vi "2_1_LV23.vi"() -> ()   [LabVIEW 2023, in "2025.lvlib"]
uses:
  2025.lvlib
  <vilib>/Analysis/NI_AALBase.lvlib
  <vilib>/Analysis/1siggen.llb/Ramp Pattern by Delta.vi
  Program Files/National Instruments/LabVIEW 2025/user.lib/_OpenG.lib/string/string.llb/openg_string.lvlib
  Program Files/National Instruments/LabVIEW 2025/user.lib/_OpenG.lib/string/string.llb/Trim Whitespace (String Array)__ogtk.vi
panel:
  out "size(s)":i32
  out "Numeric":i32
  out "sum 2":u64
  out "number 2":u64[](array[numeric])
  out "Array 2":string[](array[string])
  out "output 7":string
  out "String out":string[](array[string])
  out "output 4":string
  out "output 3":string
  in  "Boolean":bool
  out "sum":u64
  out "number":u64[](array[numeric])
  out "Array":string[](array[string])
  out "substring 2":string
  out "substring":string
  out "length":i32
  out "decimal integer string":string[](array[string])
  out "Ramp Pattern":u64[](array[numeric])
  out "output 2":i32
  out "output 1":i32
  out "array":string[](array[string])
  # "1736195310 too LOW"
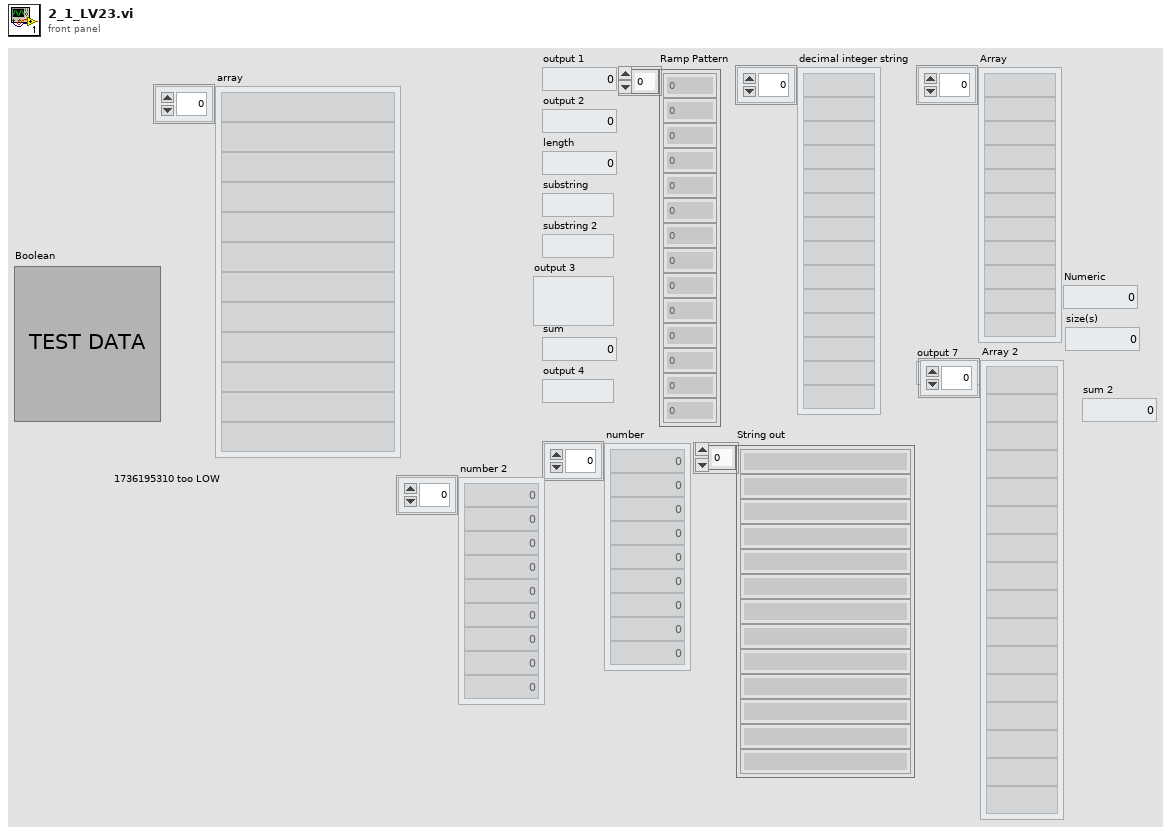
[diagram p1: front panel]
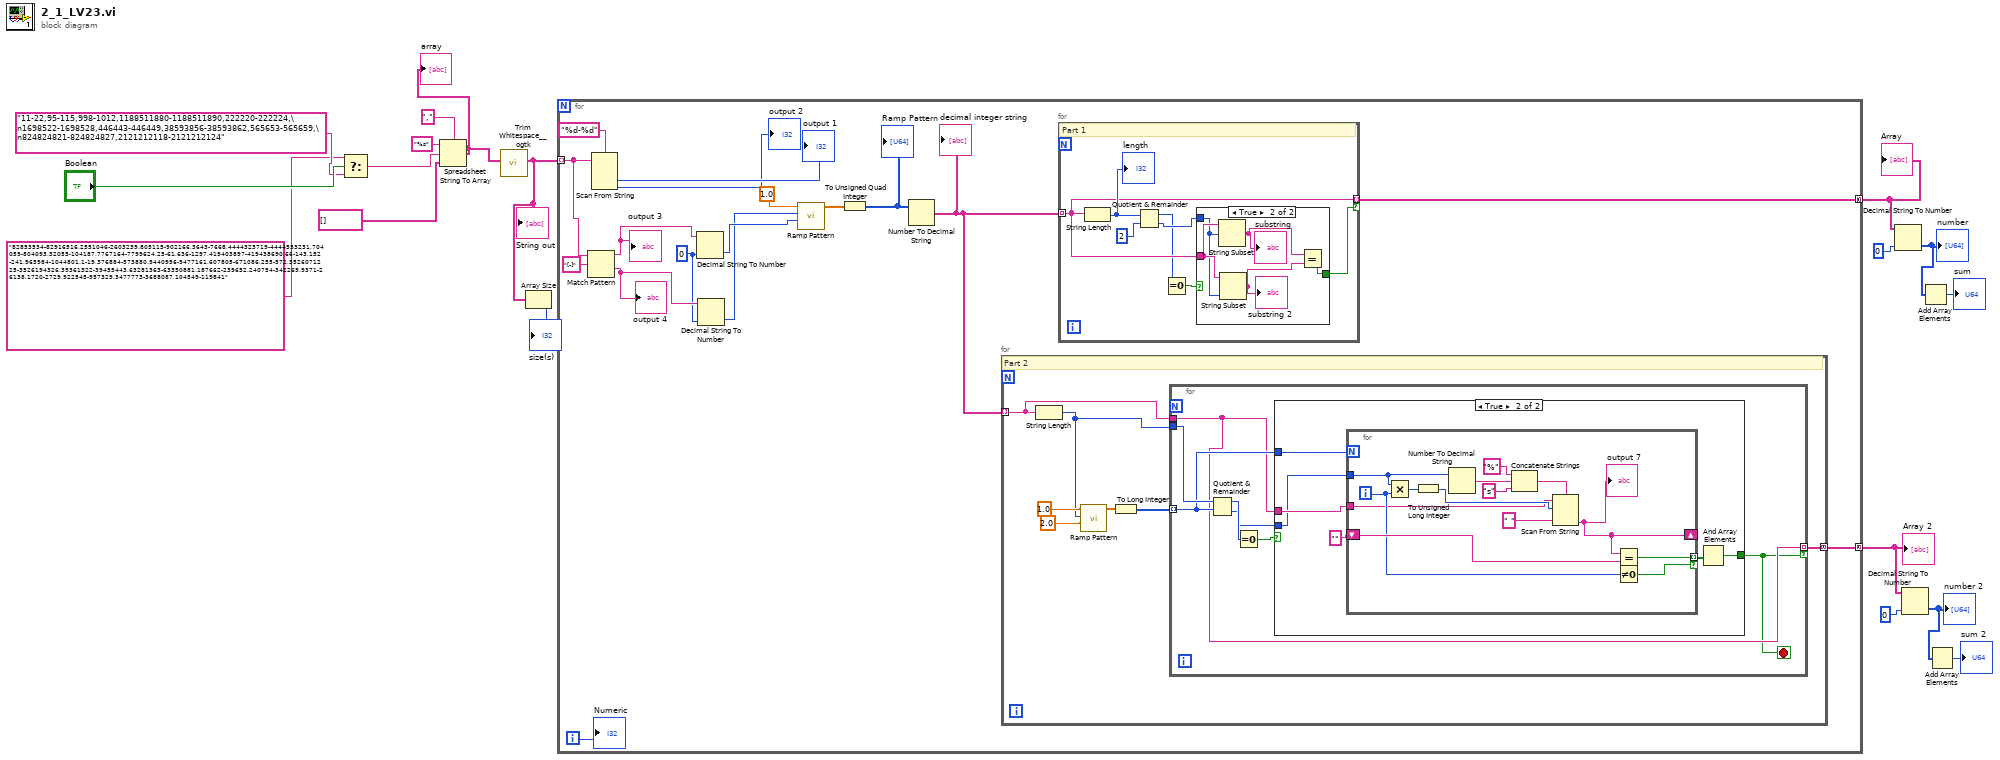
[diagram p0: block diagram]
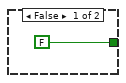
[diagram p3: hidden frame]
diagram:
  n1 = Select(t="82853534-82916516,2551046-2603239,805115-902166,3643-7668,4444323719-4444553231,704059-804093,32055-104187,7767164-7799624,25-61,636-1297,419403897-419438690,66-143,152-241,965984-1044801,1-19,376884-573880,9440956-9477161,607805-671086,255-572,3526071225-3526194326,39361322-39455443,63281363-63350881,187662-239652,240754-342269,9371-26138,1720-2729,922545-957329,3477773-3688087,104549-119841", s="Boolean", f="11-22,95-115,998-1012,1188511880-1188511890,222220-222224,\n1698522-1698528,446443-446449,38593856-38593862,565653-565659,\n824824821-824824827,2121212118-2121212124") -> (s? t:f=w8:string)
  n2 = Spreadsheet String To Array(delimiter (Tab)=",", format string="%s", spreadsheet string=w8, array type (2D Dbl)=string[] []) -> (array=w7:string[])
  "array" <- w7
  n3 = call-poly "Trim Whitespace__ogtk.vi"("String in"=w7) -> ("String out"=w2:string[])  [unwired: 6 in]
  "String out" <- w2
  n4 = Array Size(array=w2) -> (size(s)=→"size(s)":i32)
  n5 = for {
    tunnel: w2 -> [w28] mode=indexing
    tunnel: [w31] -> w15 mode=concatenating
    tunnel: [w20] -> w3 mode=concatenating
    i -> [w19]
    w24 = u64 0 ("default (0 I32)")
    n6 = Match Pattern(string=w28, regular expression="[-]") -> (before substring=w26:string, after substring=w25:string)  [unwired: 1 in, 2 out]
    "output 3" <- w26
    "output 4" <- w25
    n7 = Scan From String(format string="%d-%d", input string=w28) -> (output 1=→"output 1":i32, output 2=→"output 2":i32)  [unwired: 4 in, 3 out]
    n8 = Decimal String To Number(string=w26, default (0L)=w24) -> (number=w23:u64)  [unwired: 1 in, 1 out]
    n9 = Decimal String To Number(string=w25, default (0L)=w24) -> (number=w22:u64)  [unwired: 1 in, 1 out]
    n10 = call-poly <vilib>:"Ramp Pattern.vi"("start"=w23, "end"=w22, "delta"=1.0) -> ("Ramp Pattern"=w33:dbl[])  [unwired: 6 in, 2 out]
    n11 = To Unsigned Quad Integer(1:w33) -> (0:w32:u64[])
    "Ramp Pattern" <- w32
    n12 = Number To Decimal String(number=w32) -> (decimal integer string=w21:string[])  [unwired: 1 in]
    "decimal integer string" <- w21
    n13 = for {
      tunnel: w21 -> [w38] mode=indexing
      tunnel: [w36] -> w20 mode=concatenating
      # "Part 2"
      n14 = String Length(string=w38) -> (length=w37:i32)
      n15 = call-poly <vilib>:"Ramp Pattern.vi"("start"=2.0, "end"=w37, "delta"=1.0) -> ("Ramp Pattern"=w40:dbl[])  [unwired: 6 in, 2 out]
      n16 = To Long Integer(number=w40) -> (32bit integer=w39:i32[])
      n17 = for {
        tunnel: w39 -> [w45] mode=indexing
        tunnel: w38 -> [w44]
        tunnel: w37 -> [w49]
        tunnel: [w44] -> w36 mode=indexing if=w43
        stop <- w43 stop-if-true
        n18 = Quotient & Remainder(x=w49, y=w45) -> (x-y*floor(x/y)=w47:i32, floor(x/y)=w46:i32)
        n19 = Equal To 0?(x=w47) -> (x = 0?=w48:bool)
        n20 = case shown="True" w48 {
          tunnel: w46 -> [_ w54]
          tunnel: w44 -> [_ w55]
          tunnel: w45 -> [_ w53]
          tunnel: [_ w50] -> w43
          frame False {
          }
          frame True {
            n21 = for {
              N: w53 -> [_]
              tunnel: w54 -> [w62]
              tunnel: w55 -> [w56]
              shift-right: [w61] -> _
              shift-left: "" ("format string") -> [w60]
              tunnel: [w58] -> w51 mode=indexing if=w57
              i -> [w59]
              n22 = Multiply(x=w62, y=w59) -> (x*y=w69:i32)
              n23 = To Unsigned Long Integer(number=w69) -> (unsigned 32bit integer=w64:u32)
              n24 = Number To Decimal String(number=w62) -> (decimal integer string=w65:string)  [unwired: 1 in]
              n25 = Concatenate Strings("%" ("format string"), w65, "s" ("format string")) -> (w68:string)
              n26 = Scan From String(format string=w68, input string=w56, initial scan location=w64, default 1=" " ("format string")) -> (output 1=w61:string)  [unwired: 1 in, 3 out]
              "output 7" <- w61
              n27 = Equal?(x=w61, y=w60) -> (x = y?=w58:bool)
              n28 = Not Equal To 0?(x=w59) -> (x != 0?=w57:bool)
            }
            n29 = And Array Elements(Boolean array=w51) -> (logical AND=w50:bool)
          }
        }
      }
    }
    n30 = for {
      tunnel: w21 -> [w74] mode=indexing
      tunnel: [w74] -> w31 mode=indexing if=w72
      # "Part 1"
      n31 = String Length(string=w74) -> (length=w75:i32)
      "length" <- w75
      n32 = Quotient & Remainder(x=w75, y=2) -> (x-y*floor(x/y)=w70:i32, floor(x/y)=w71:i32)
      n33 = Equal To 0?(x=w70) -> (x = 0?=w73:bool)
      n34 = case shown="True" w73 {
        tunnel: w74 -> [_ w82]
        tunnel: w71 -> [_ w81]
        tunnel: [FALSE w78] -> w72
        frame False {
        }
        frame True {
          n35 = String Subset(string=w82, offset (0)=w81) -> (substring=w80:string)  [unwired: 1 in]
          "substring" <- w80
          n36 = String Subset(string=w82, length (rest)=w81) -> (substring=w79:string)  [unwired: 1 in]
          "substring 2" <- w79
          n37 = Equal?(x=w80, y=w79) -> (x = y?=w78:bool)
        }
      }
    }
    "Numeric" <- w19
  }
  "Array" <- w15
  "Array 2" <- w3
  n38 = Decimal String To Number(string=w15, default (0L)=u64 0 ("default (0 I32)")) -> (number=w14:u64[])  [unwired: 1 in, 1 out]
  "number" <- w14
  n39 = Decimal String To Number(string=w3, default (0L)=u64 0 ("default (0 I32)")) -> (number=w6:u64[])  [unwired: 1 in, 1 out]
  "number 2" <- w6
  n40 = Add Array Elements(numeric array=w14) -> (sum=→"sum":u64)
  n41 = Add Array Elements(numeric array=w6) -> (sum=→"sum 2":u64)
